vi "Auto_indexing_array.vi"() -> ()   [LabVIEW 2019]
panel:
  out "Array\nElements":dbl
  in  "Input\n Array":dbl[](array[numeric])
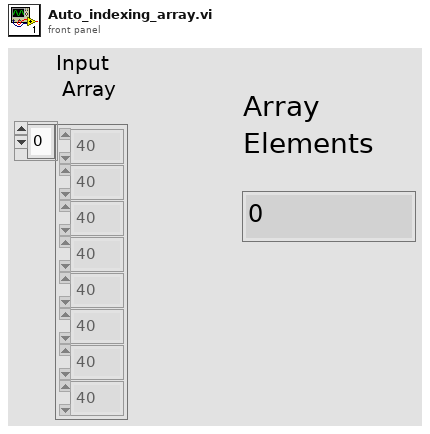
[diagram p1: front panel]
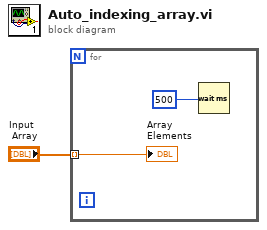
[diagram p0: block diagram]
diagram:
  n1 = for {
    tunnel: "Input\n Array" -> [w2] mode=indexing
    n2 = Wait (ms)(milliseconds to wait=u32 500) -> ()  [unwired: 1 out]
    "Array\nElements" <- w2
  }
